vi "_generateProfilePath.vi"(6 "profileImport":T1[](array[typedef]), 8 "error in (no error)":errorcluster, 10 "Target?":bool, 11 "OSArch":string) -> (0 "error out":errorcluster, 1 "result out":i32[](array[numeric]), 2 "profileDestPath":string[](array[string]), 3 "profileSrcPath":string[](array[string]))   [LabVIEW 2020, in "SEECD System Explorer.lvlib"]
uses:
  SEECD System Explorer.lvlib
  <resource>/Framework/Providers/indcomecat/_InternalSubVIs/_profileImport.ctl
  Applications/Utilities/ECAT Files.ctl
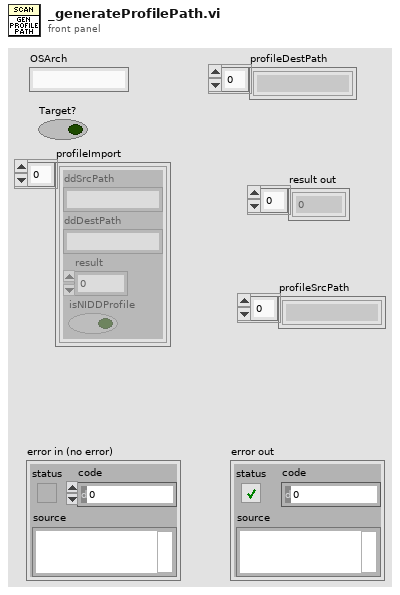
[diagram p1: front panel]
types:
  T1 = typedef "_profileImport.ctl" = cluster{"ddSrcPath":string, "ddDestPath":string, "result":i32, "isNIDDProfile":bool}
  T2 = typedef "SEECD System Explorer.lvlib/ECAT Files.ctl" = enum16{"niECATLVProvider.mxx", "indcomecat.chm", "Providers DD", "Shared DD"}
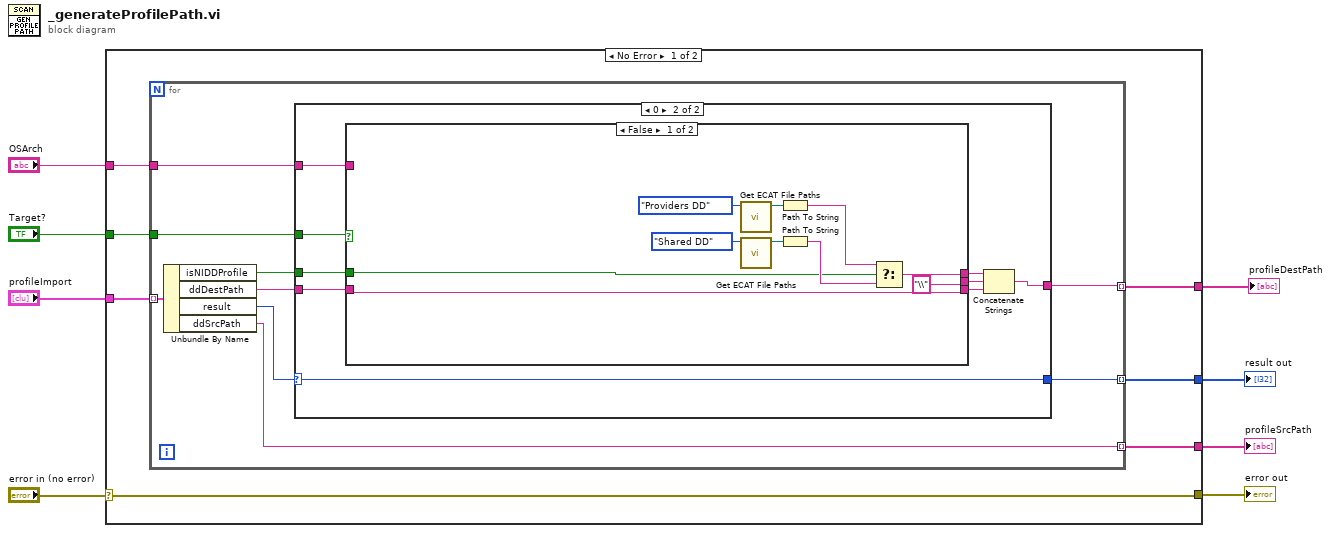
[diagram p0: block diagram]
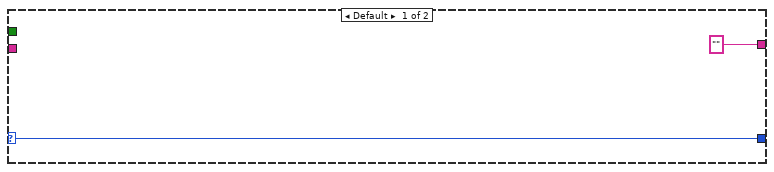
[diagram p2: hidden frame]
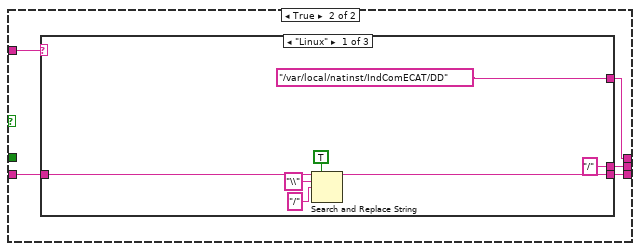
[diagram p3: hidden frame]
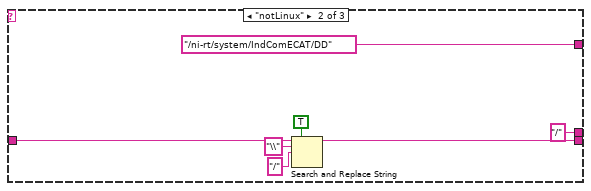
[diagram p4: hidden frame]
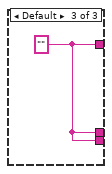
[diagram p5: hidden frame]
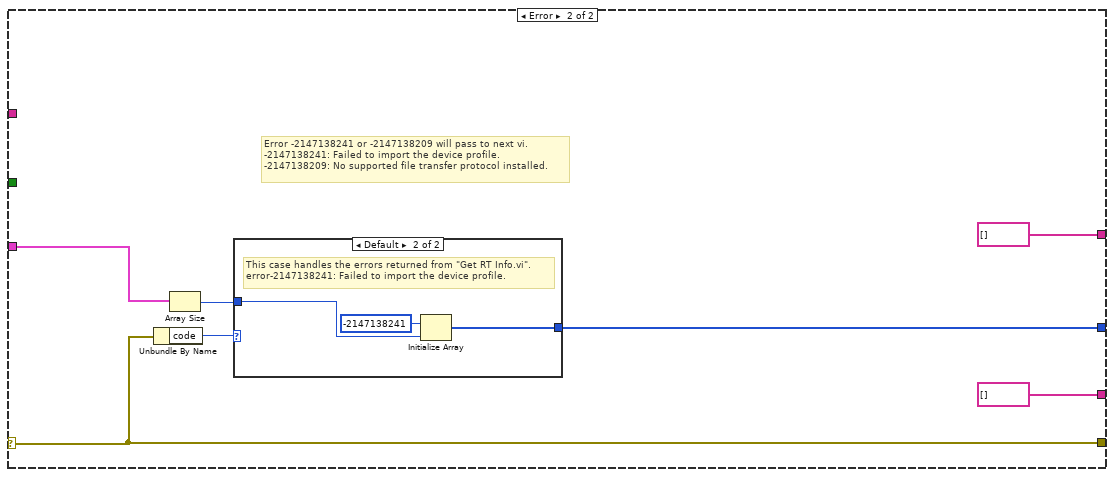
[diagram p6: hidden frame]
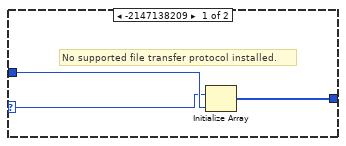
[diagram p7: hidden frame]
diagram:
  n1 = case shown="No Error" "error in (no error)" {
    selector: "error in (no error)" -> [w14 w70]
    tunnel: [w15 string[] []] -> w8
    tunnel: "OSArch" -> [w10 _]
    tunnel: [w14 w70] -> w6
    tunnel: [w13 w66] -> w5
    tunnel: "profileImport" -> [w12 w68]
    tunnel: [w11 string[] []] -> w4
    tunnel: "Target?" -> [w9 _]
    frame No Error {
      n2 = for {
        tunnel: [w24] -> w15 mode=indexing
        tunnel: [w23] -> w13 mode=indexing
        tunnel: w12 -> [w22] mode=indexing
        tunnel: [w19] -> w11 mode=indexing
        tunnel: w10 -> [w17]
        tunnel: w9 -> [w16]
        n3 = Unbundle By Name(w22) -> ("isNIDDProfile"=w18:bool, "ddDestPath"=w20:string, "result"=w21:i32, "ddSrcPath"=w19:string)
        n4 = case shown="0" w21 {
          selector: w21 -> [w25 w35]
          tunnel: w18 -> [_ w34]
          tunnel: w20 -> [_ w32]
          tunnel: ["" ("result string") w30] -> w24
          tunnel: [w25 w35] -> w23
          tunnel: w17 -> [_ w33]
          tunnel: w16 -> [_ w27]
          frame Default {
          }
          frame 0 {
            n5 = case shown="False" w27 {
              tunnel: w34 -> [w40 _]
              tunnel: w33 -> [_ w50]
              tunnel: w32 -> [w42 w49]
              tunnel: [w42 w48] -> w31
              tunnel: [w41 w47] -> w29
              tunnel: ["\\" w46] -> w28
              frame False {
                n6 = call "Get ECAT File Paths.vi"("ECAT File"=ECAT_Files."Providers DD") -> ("File Path"=w37:path)  [unwired: 9 in, 1 out]
                n7 = call "Get ECAT File Paths.vi"("ECAT File"=ECAT_Files."Shared DD") -> ("File Path"=w36:path)  [unwired: 9 in, 1 out]
                n8 = Path To String(path=w37) -> (string=w45:string)
                n9 = Path To String(path=w36) -> (string=w44:string)
                n10 = Select(t=w45, s=w40, f=w44) -> (s? t:f=w41:string)
              }
              frame True {
                n11 = case shown="\"Linux\"" w50 {
                  tunnel: ["/var/local/natinst/IndComECAT/DD" "/ni-rt/system/IndComECAT/DD" w65] -> w47
                  tunnel: w49 -> [w53 w59 _]
                  tunnel: [w52 w58 w65] -> w48
                  tunnel: ["/" "/" w65] -> w46
                  frame "Linux" {
                    n12 = Search and Replace String(replace all?=TRUE ("replace all? (F)"), input string=w53, search string="\\", replace string="/" ("replace string (\"\")")) -> (result string=w52:string)  [unwired: 4 in, 3 out]
                  }
                  frame "notLinux" {
                    n13 = Search and Replace String(replace all?=TRUE ("replace all? (F)"), input string=w59, search string="\\", replace string="/" ("replace string (\"\")")) -> (result string=w58:string)  [unwired: 4 in, 3 out]
                  }
                  frame Default {
                    w65 = ""
                  }
                }
              }
            }
            n14 = Concatenate Strings(w29, w28, w31) -> (w30:string)
          }
        }
      }
    }
    frame Error {
      # "Error -2147138241 or -2147138209 will pass to next vi.\n-2147138241: Failed to import the device profile.\n-2147138209: No supported file transfer protocol installed."
      n15 = Unbundle By Name(w70) -> ("code"=w69:i32)
      n16 = Array Size(array=w68) -> (size(s)=w67:i32)
      n17 = case shown="Default" w69 {
        selector: w69 -> [w73 _]
        tunnel: [w75 w77] -> w66
        tunnel: w67 -> [w74 w78]
        frame -2147138209 {
          # "No supported file transfer protocol installed."
          n18 = Initialize Array(w73, w74) -> (w75:i32[])
        }
        frame Default {
          # "This case handles the errors returned from \"Get RT Info.vi\".\nerror-2147138241: Failed to import the device profile."
          n19 = Initialize Array(-2147138241 ("element"), w78) -> (w77:i32[])
        }
      }
    }
  }
  "profileDestPath" <- w8
  "error out" <- w6
  "result out" <- w5
  "profileSrcPath" <- w4
